vi "Reset-180to180Angle.vi"(10 "Offset":dbl, 11 "AngleInput":dbl) -> (3 "AngleOutput":dbl)   [LabVIEW 2018]
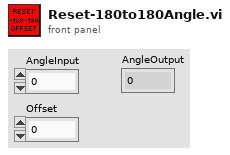
[diagram p1: front panel]
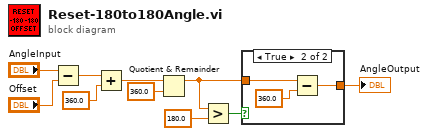
[diagram p0: block diagram]
diagram:
  n1 = Subtract(x="AngleInput", y="Offset") -> (x-y=w8:dbl)
  n2 = Add(x=w8, y=360.0) -> (x+y=w6:dbl)
  n3 = Quotient & Remainder(x=w6, y=360.0) -> (x-y*floor(x/y)=w2:dbl)  [unwired: 1 out]
  n4 = Greater?(x=w2, y=180.0) -> (0:w4:bool)
  n5 = case shown="True" w4 {
    tunnel: w2 -> [w11 w13]
    tunnel: [w11 w12] -> w1
    frame False {
    }
    frame True {
      n6 = Subtract(x=w13, y=360.0) -> (x-y=w12:dbl)
    }
  }
  "AngleOutput" <- w1
